vi "SwissSPAD Live_Abort Saving Tasks.vi"(8 "Error In":errorcluster) -> (0 "Error Out":errorcluster, 2 "Notebook Message":string, 3 "UI Message":string)   [LabVIEW 2021]
uses:
  SwissSPAD Live_Internal Data List.ctl
  SwissSPAD Live_File Saving Task Information.ctl
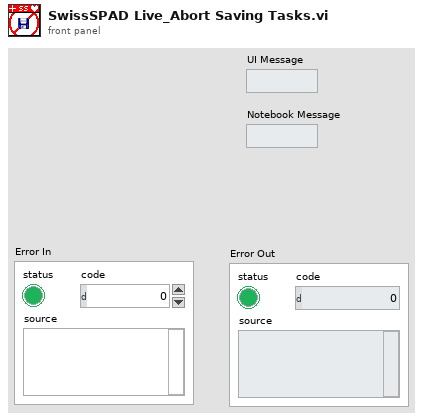
[diagram p1: front panel]
types:
  T1 = typedef "SwissSPAD Live_File Saving Task Information.ctl" = cluster{"File Path::n":string, "# Saved Images":i32, "# Images (Total)":i32, "File Size (Bytes)":i64}
  T2 = typedef "SwissSPAD Live_Internal Data List.ctl" = enum16{"Number of pending file saving tasks", "File Saving Tasks Information", "Current Image ROI Information", "# FPGA Reset Attempts", "Histogram Cursor Locations", "Histogram Window is Open"}
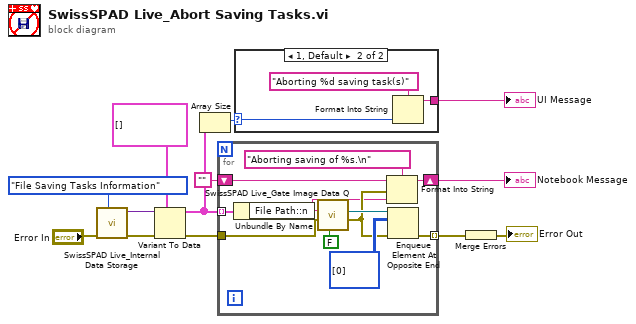
[diagram p0: block diagram]
diagram:
  n1 = call "SwissSPAD Live_Internal Data Storage.vi"("SS2 Live Data"=SwissSPAD_Live_Internal_Data_List."File Saving Tasks Information", "Error In"="Error In") -> ("Error Out"=w11:errorcluster, "Variant"=w12:variant)  [unwired: 7 in, 1 out]
  n2 = Variant To Data(error in=w11, type=T1[] [] ("Array"), Variant=w12) -> (data=w3:T1[], error out=w8:errorcluster)
  n3 = Array Size(array=w3) -> (size(s)=w2:i32)
  n4 = for {
    tunnel: w3 -> [w24] mode=indexing
    tunnel: w8 -> [w23]
    tunnel: [w20] -> w7 mode=indexing
    shift-right: [w18] -> w4
    shift-left: "" -> [w19]
    n5 = Unbundle By Name(w24) -> ("File Path::n"=w16:string)
    n6 = call "SwissSPAD Live_Gate Image Data Q.vi"("create if not found? (T)"=FALSE, "error in (no error)"=w23, "SwissSPAD Live Gate Image Data Q Name"=w16) -> ("error out"=w17:errorcluster, "SwissSPAD Live Gate Image Data Q"=w22:refnum<queue>)  [unwired: 6 in, 1 out]
    n7 = Format Into String(format string="Aborting saving of %s.\n", initial string=w19, error in=w17, w16) -> (resulting string=w18:string)  [unwired: 1 out]
    n8 = Enqueue Element At Opposite End(queue=w22, element=u8[][] [[0]], error in (no error)=w17) -> (error out=w20:errorcluster)  [unwired: 1 in, 2 out]
  }
  "Notebook Message" <- w4
  n9 = case shown="1, Default" w2 {
    selector: w2 -> [_ w25]
    tunnel: [_ w27] -> w1
    frame 0 {
    }
    frame 1, Default {
      n10 = Format Into String(format string="Aborting %d saving task(s)" ("UI Message"), w25) -> (resulting string=w27:string)  [unwired: 2 in, 1 out]
    }
  }
  "UI Message" <- w1
  n11 = Merge Errors(w7) -> (→"Error Out":errorcluster)
